vi "NIClearErrors.vi"(8 "error in (no error)":errorcluster, 11 "Motion Settings":T1={"No Motion?"=FALSE, "Motion System"=enum."NI 735x", "Motion Bd ID"=1, "Motion Profile"="SMAC1", "# Axis"=1, "Reverse Z axis?"=TRUE, "SMAC Axis"=0, "scan pair"=enum."y-(x) scan", "RT fps"=6.0, "Steps per mm"=[1000, 1000, 1000, 1000], "Motor Parameters"={"velocity ct/s"=[10000.0, 10000.0, 10000.0, 50000.0], "accel ct/s^2"=[50000.0, 50000.0, 50000.0, 200000.0]}, "One Way Scan"=FALSE, "Reverse One Way Scan"=FALSE, "Global Position (mm)"=[], "Plane"=0, "Distance between\nscan lines (um)"=0.0, "Distance between\nscan planes (um)"=0.0, "number of scan planes"=1, "Total steps in line"=0, "Xtra plane\ndistance  (um)"=100, "Xtra planes "=1, "Add Axis"=FALSE, "overshoot cts"=200, "BKPT Shift"=0, "Scan Start Time (ms)"=0, "ESP VISA"="GPIB::1::INSTR", "3rd Axis"=1, "GL Ref Out"=refnum, "Galil Address"=""} {"3rd Axis" items=["x", "y", "z", "w"]; "Xtra planes" min=1; "Xtra plane\ndistance  (um)" min=0; "Distance between\nscan planes (um)" format="%.2f"; "Distance between\nscan lines (um)" format="%.2f"; "SMAC Axis" items=["None"=0, "Axis 1"=1, "Axis 2"=2, "Axis 3"=3, "Axis 4"=4, "Axis 5"=5, "Axis 6"=6, "Axis 7"=7, "Axis 8"=8, "Vector Space 1"=17, "Vector Space 2"=18, "Vector Space 3"=19, "Vector Space 4"=20]; "Motion Bd ID" min=1 max=32 step=1}) -> (0 "error out":errorcluster, 2 "Error?":bool, 3 "Motion Settings Out":T1={"No Motion?"=FALSE, "Motion System"=enum."NI 735x", "Motion Bd ID"=1, "Motion Profile"="SMAC1", "# Axis"=1, "Reverse Z axis?"=TRUE, "SMAC Axis"=0, "scan pair"=enum."y-(x) scan", "RT fps"=6.0, "Steps per mm"=[1000, 1000, 1000, 1000], "Motor Parameters"={"velocity ct/s"=[10000.0, 10000.0, 10000.0, 50000.0], "accel ct/s^2"=[50000.0, 50000.0, 50000.0, 200000.0]}, "One Way Scan"=FALSE, "Reverse One Way Scan"=FALSE, "Global Position (mm)"=[], "Plane"=0, "Distance between\nscan lines (um)"=0.0, "Distance between\nscan planes (um)"=0.0, "number of scan planes"=1, "Total steps in line"=0, "Xtra plane\ndistance  (um)"=100, "Xtra planes "=1, "Add Axis"=FALSE, "overshoot cts"=200, "BKPT Shift"=0, "Scan Start Time (ms)"=0, "ESP VISA"="GPIB::1::INSTR", "3rd Axis"=1, "GL Ref Out"=refnum, "Galil Address"=""} {"3rd Axis" items=["x", "y", "z", "w"]; "Xtra planes" min=1; "Xtra plane\ndistance  (um)" min=0; "Distance between\nscan planes (um)" format="%.2f"; "Distance between\nscan lines (um)" format="%.2f"; "SMAC Axis" items=["None"=0, "Axis 1"=1, "Axis 2"=2, "Axis 3"=3, "Axis 4"=4, "Axis 5"=5, "Axis 6"=6, "Axis 7"=7, "Axis 8"=8, "Vector Space 1"=17, "Vector Space 2"=18, "Vector Space 3"=19, "Vector Space 4"=20]; "Motion Bd ID" min=1 max=32 step=1})   [LabVIEW 2022 SP3]
uses:
  MotionParameters.ctl
  MotionSys.ctl
  -MotionRoutines/ScanAxis.ctl
  -MotionRoutines/3rdAxis.ctl
panel:
  # "1-D and 2-D B scan settings"
  # "1-D and 2-D B scan settings"
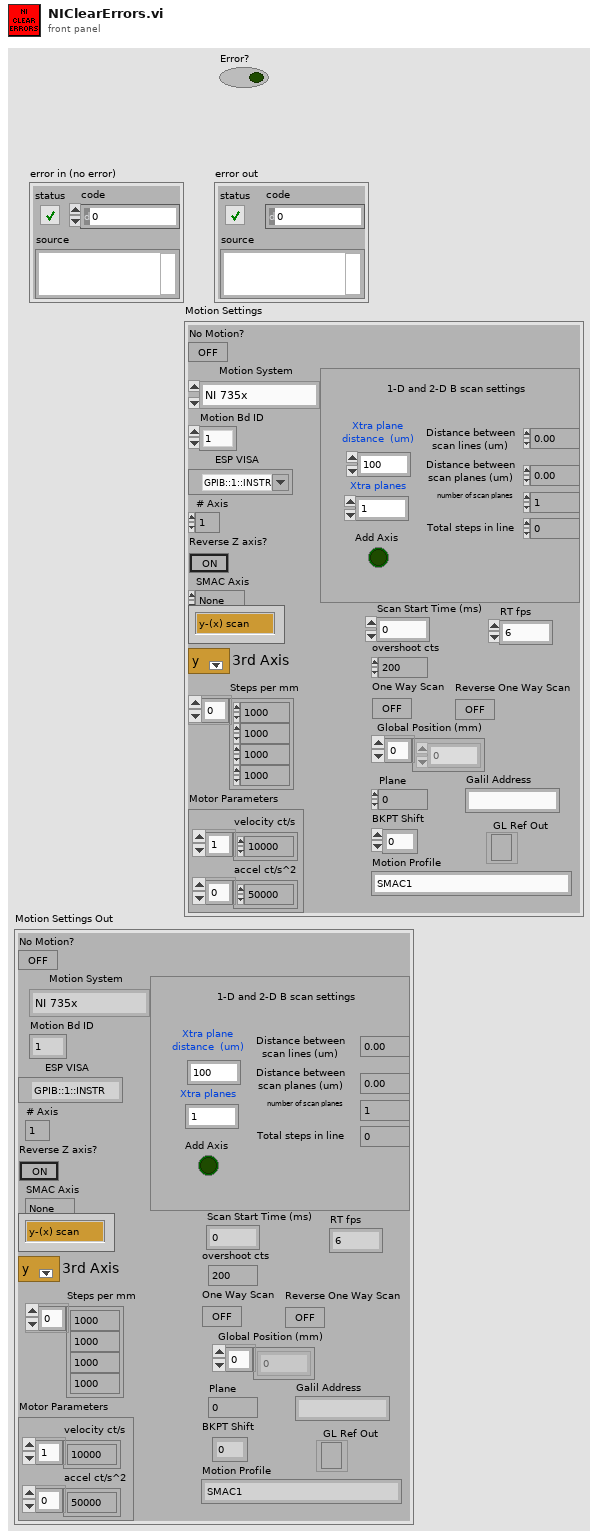
[diagram p1: front panel]
types:
  T1 = typedef "MotionParameters.ctl" = cluster{"No Motion?":bool, "Motion System":T2, "Motion Bd ID":u8, "Motion Profile":string, "# Axis":i8, "Reverse Z axis?":bool, "SMAC Axis":u16, "scan pair":T3, "RT fps":sgl, "Steps per mm":i32[], "Motor Parameters":cluster{"velocity ct/s":dbl[], "accel ct/s^2":dbl[]}, "One Way Scan":bool, "Reverse One Way Scan":bool, "Global Position (mm)":dbl[], "Plane":i32, "Distance between\nscan lines (um)":sgl, "Distance between\nscan planes (um)":sgl, "number of scan planes":i32, "Total steps in line":i32, "Xtra plane\ndistance  (um)":i32, "Xtra planes ":i32, "Add Axis":bool, "overshoot cts":i32, "BKPT Shift":i32, "Scan Start Time (ms)":u32, "ESP VISA":refnum<visa-resource-name>, "3rd Axis":T4, "GL Ref Out":refnum<k7>, "Galil Address":string}
  T2 = typedef "MotionSys.ctl" = enum16{"MM3000", "NI 735x", "Newport ESP", "No Motion Card", "Galil"}
  T3 = typedef "ScanAxis.ctl" = enum16{"y-(x) scan", "x-(y) scan", "z-(x) scan", "z-(y) scan", "y-(z) scan", "x-(z) scan", "w-(x) scan", "w-(y) scan", "w-(z) scan", "x-(w) scan", "y-(w) scan", "z-(w) scan"}
  T4 = typedef "3rdAxis.ctl" = u16
  T5 = typedef "Bd Id Out" = u8
  T6 = cluster{"Ready to Receive":bool, "Return Data Pending":bool, "Reserved":bool, "CIP":bool, "Packet Error":bool, "Power Up Reset":bool, "Error Message":bool, "Hardware Fail":bool}
  T7 = typedef "BoardID.ctl" = i32
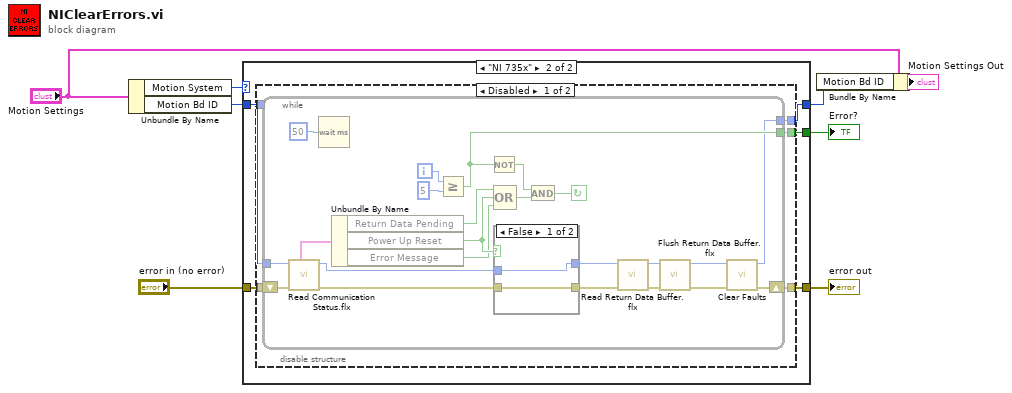
[diagram p0: block diagram]
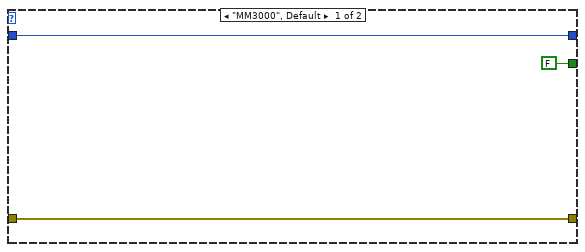
[diagram p2: hidden frame]
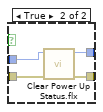
[diagram p3: hidden frame]
diagram:
  n1 = Unbundle By Name("Motion Settings") -> ("Motion System"=w5:T2, "Motion Bd ID"=w4:u8)
  n2 = case shown="\"NI 735x\"" w5 {
    tunnel: [FALSE w16] -> w8
    tunnel: [w9 w15] -> w7
    tunnel: [w10 w14] -> w1
    tunnel: "error in (no error)" -> [w9 w13]
    tunnel: w4 -> [w10 w12]
    frame "MM3000", Default {
    }
    frame "NI 735x" {
      n3 = disable-structure shown="Disabled" {
        disable-tunnel: [w21 _] -> w16
        disable-tunnel: [w20 _] -> w15
        disable-tunnel: [w19 _] -> w14
        disable-tunnel: w13 -> [w18 _]
        disable-tunnel: w12 -> [w17 _]
        frame Disabled {
          n4 = while {
            tunnel: w17 -> [w44]
            tunnel: [w25] -> w19
            shift-right: [w27] -> w20
            shift-left: w18 -> [w41]
            tunnel: [w30] -> w21
            i -> [w33]
            stop <- w32 continue-if-true
            n5 = call <vilib>:"Read Communication Status.flx"("error in (no error)"=w41, "Board ID"=w44) -> ("error out"=w40:errorcluster, "Bd ID Out"=w42:T5, "Communication Status Register"=w43:T6)  [unwired: 4 in]
            n6 = Wait (ms)(milliseconds to wait=u32 50) -> ()  [unwired: 1 out]
            n7 = Unbundle By Name(w43) -> ("Return Data Pending"=w36:bool, "Power Up Reset"=w37:bool, "Error Message"=w24:bool)
            n8 = Greater Or Equal?(x=w33, y=5) -> (x >= y?=w30:bool)
            n9 = Not(x=w30) -> (.not. x?=w29:bool)
            n10 = Compound Arithmetic op=OR(w36, w37, w24) -> (w31:bool)
            n11 = case shown="False" w37 {
              tunnel: w42 -> [w46 w50]
              tunnel: [w46 w49] -> w39
              tunnel: w40 -> [w45 w48]
              tunnel: [w45 w47] -> w38
              frame False {
              }
              frame True {
                n12 = call <vilib>:"Clear Power Up Status.flx"("error in (no error)"=w48, "Board ID"=w50) -> ("error out"=w47:errorcluster, "Bd ID Out"=w49:T5)  [unwired: 5 in]
              }
            }
            n13 = And(x=w29, y=w31) -> (x .and. y?=w32:bool)
            n14 = call <vilib>:"Read Return Data Buffer.flx"("error in (no error)"=w38, "Board ID"=w39) -> ("error out"=w22:errorcluster, "Bd ID Out"=w23:T5)  [unwired: 4 in, 4 out]
            n15 = call <vilib>:"Flush Return Data Buffer.flx"("error in (no error)"=w22, "Board ID"=w23) -> ("error out"=w28:errorcluster, "Bd ID Out"=w26:T5)  [unwired: 5 in]
            n16 = call <vilib>:"Clear Faults.vi"("error in (no error)"=w28, "board in"=w26) -> ("error out"=w27:errorcluster, "board out"=w25:T7)  [unwired: 8 in]
          }
        }
        frame Enabled {
        }
      }
    }
  }
  "Error?" <- w8
  "error out" <- w7
  n17 = Bundle By Name(cluster="Motion Settings", "Motion Bd ID"=w1) -> (→"Motion Settings Out":T1)
